vi "Write Condition.vi"(10 "Deny":u16[](array[numeric]), 11 "IL U16 Deny in":refnum<class "IL U16 Seize.lvclass">) -> (3 "IL U16 Deny out":refnum<class "IL U16 Seize.lvclass">)   [LabVIEW 2015, in "Interlocks.lvlib" / "IL U16 Seize.lvclass"]
uses:
  IL U16 Seize.lvclass
  IL U16 Seize.lvclass/IL U16 Seize.ctl
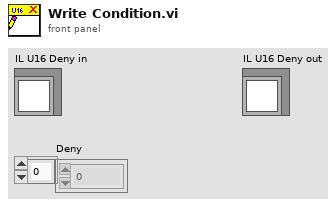
[diagram p1: front panel]
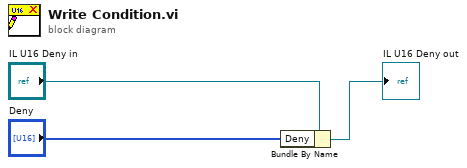
[diagram p0: block diagram]
diagram:
  n1 = Bundle By Name(cluster="IL U16 Deny in", "Deny"="Deny") -> (→"IL U16 Deny out":refnum<class "IL U16 Seize.lvclass">)
